vi "RegisterTrendPointsRoutedMessage_Parse.vi"(8 "error in (no error)":errorcluster, 11 "message":variant) -> (0 "error out":errorcluster, 2 "RegisterTrend":T1)   [LabVIEW 2017, in "DataEventCreator.lvlib"]
uses:
  <vilib>/addons/InsightCM/Devices/Shared/Common/DataEventCreator/DataEventCreator.lvlib
  <vilib>/addons/InsightCM/Devices/Shared/Common/DataEventCreator/controls/RegisterTrendPoints.ctl
  <vilib>/addons/InsightCM/Devices/Shared/Common/DataEventCreator/controls/Registry_Trend.ctl
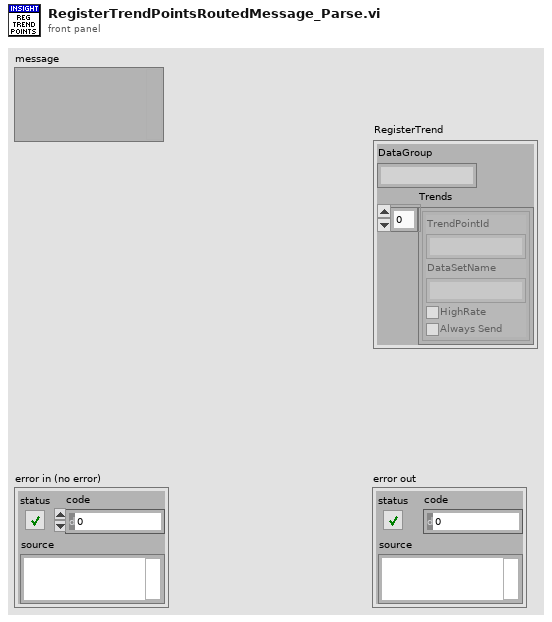
[diagram p1: front panel]
types:
  T1 = typedef "DataEventCreator.lvlib/RegisterTrendPoints.ctl" = cluster{"DataGroup":string, "Trends":T2[]}
  T2 = typedef "DataEventCreator.lvlib/Registry_Trend.ctl" = cluster{"TrendPointId":string, "DataSetName":string, "HighRate":bool, "Always Send":bool}
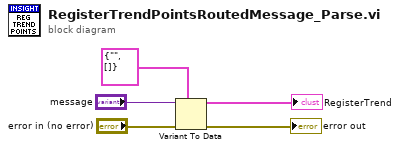
[diagram p0: block diagram]
diagram:
  n1 = Variant To Data(error in="error in (no error)", type=T1 {"DataGroup"="", "Trends"=[]} ("RegisterTrend"), Variant="message") -> (data=→"RegisterTrend":T1, error out=→"error out":errorcluster)
